vi "Is Grave.vi"(8 "Error In":errorcluster, 11 "GObject In":refnum<vi>) -> (0 "Error Out":errorcluster, 2 "Grave?":bool, 3 "GObject Out":refnum<vi>)   [LabVIEW 2017, in "Toolkit.lvlib"]
doc: "Checks if a GObject is a grave. A grave is Disable Structure with a \"Diagram Disable Structure\" style and a label that starts with \"#RIP\"."
uses:
  Toolkit.lvlib
  Typedefs/Bookmark Tags.ctl
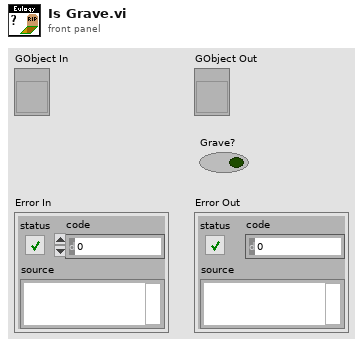
[diagram p1: front panel]
types:
  T1 = typedef "Toolkit.lvlib/Bookmark Tags.ctl" = enum16{"RIP", "Zombie"}
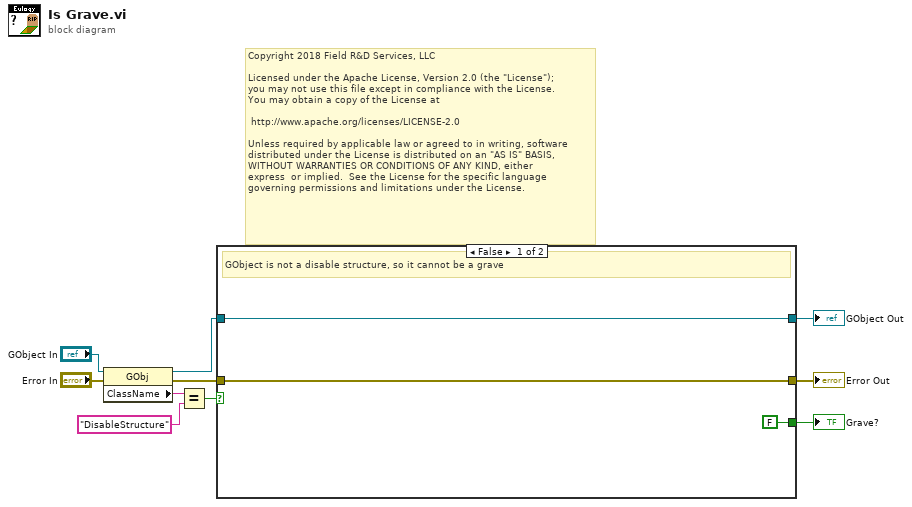
[diagram p0: block diagram]
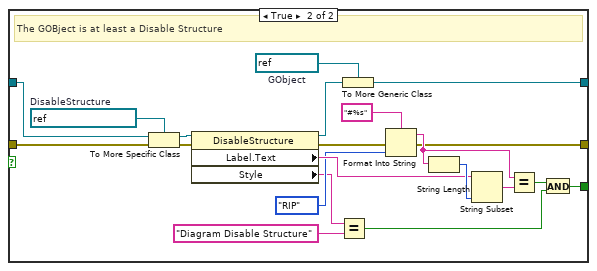
[diagram p2: hidden frame]
diagram:
  # "Copyright 2018 Field R&D Services, LLC\n\nLicensed under the Apache License, Version 2.0 (the \"License\");\nyou may not use this file except in compliance with the License.\nYou may obtain a copy of the License at\n\n\thttp://www.apache.org/licenses/LICENSE-2.0\n\nUnless required by applicable law or agreed to in writing, software\ndistributed under the License is distributed on an \"AS IS\" BASIS,\nWITHOUT WARRANTIES OR CONDITIONS OF ANY KIND, either \nexpress  or implied.  See the License for the specific language \ngoverning permissions and limitations under the License."
  n1 = property class="GObj"(reference="GObject In", error in="Error In") -> (reference out=w8:refnum<vi>, error out=w6:errorcluster, "ClassName"=w5:string)
  n2 = Equal?(x=w5, y="DisableStructure") -> (x = y?=w3:bool)
  n3 = case shown="False" w3 {
    tunnel: [FALSE w23] -> w9
    tunnel: w8 -> [w11 w20]
    tunnel: w6 -> [w13 w22]
    tunnel: [w13 w17] -> w2
    tunnel: [w11 w15] -> w1
    frame False {
      # "GObject is not a disable structure, so it cannot be a grave"
    }
    frame True {
      w14 = refnum<vi> refnum  # GObject
      w18 = refnum<vi> refnum  # DisableStructure
      # "The GOBject is at least a Disable Structure"
      n4 = To More Specific Class(target class=w18, reference=w20, error in=w22) -> (specific class reference=w19:refnum<vi>, error out=w21:errorcluster)
      n5 = property class="DisableStructure"(reference=w19, error in=w21) -> (reference out=w16:refnum<vi>, error out=w28:errorcluster, "Label.Text"=w32:string, "Style"=w27:string)
      n6 = Equal?(x=w27, y="Diagram Disable Structure") -> (x = y?=w24:bool)
      n7 = To More Generic Class(target class=w14, reference=w16) -> (generic class reference=w15:refnum<vi>)
      n8 = Format Into String(format string="#%s", error in=w28, Bookmark_Tags."RIP" ("Bookmark")) -> (resulting string=w31:string, error out=w17:errorcluster)  [unwired: 1 in]
      n9 = String Length(string=w31) -> (length=w33:i32)
      n10 = String Subset(string=w32, length (rest)=w33) -> (substring=w34:string)  [unwired: 1 in]
      n11 = Equal?(x=w31, y=w34) -> (x = y?=w25:bool)
      n12 = And(x=w25, y=w24) -> (x .and. y?=w23:bool)
    }
  }
  "Grave?" <- w9
  "GObject Out" <- w1
  "Error Out" <- w2
